vi "Load Selection.vi"() -> ()   [LabVIEW 2020]
panel:
  in  "stop":bool
  in  "12kW Load Bank with 10 Step Control":bool
  in  "1kW Load Bank with 6 Step Control":bool
  # "IoT Programmable Variable Resistive Load Bank"
  # "Select Required Capacity of Load"
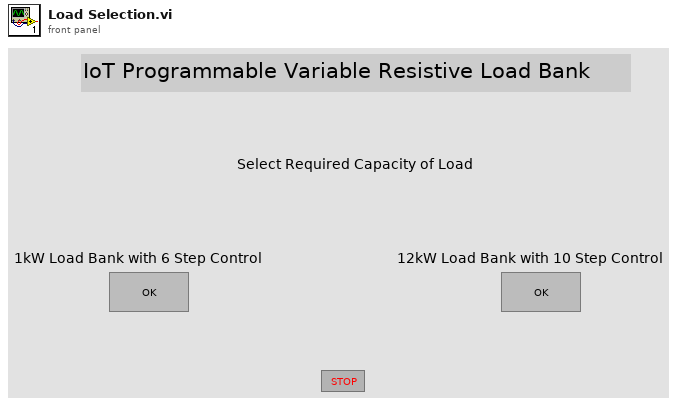
[diagram p1: front panel]
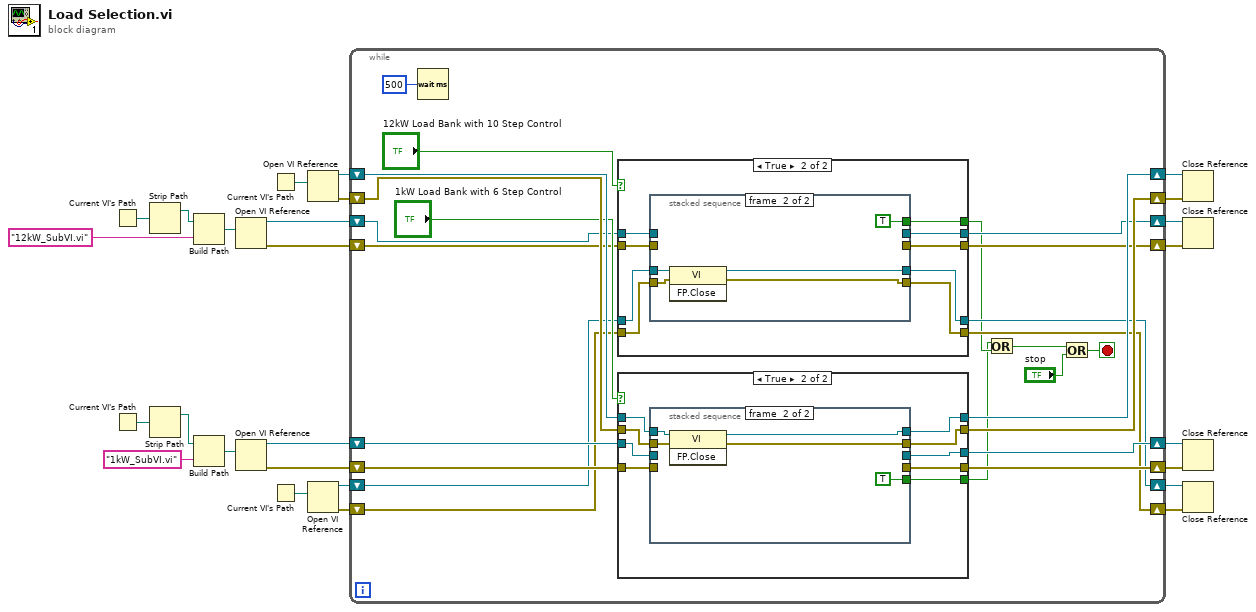
[diagram p0: block diagram]
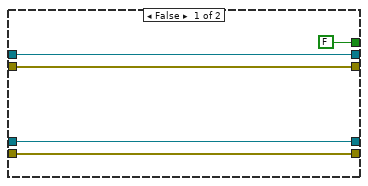
[diagram p2: hidden frame]
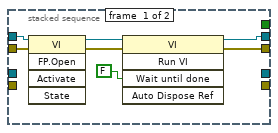
[diagram p3: hidden frame]
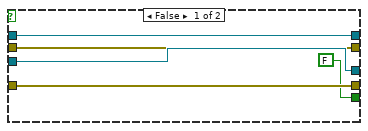
[diagram p4: hidden frame]
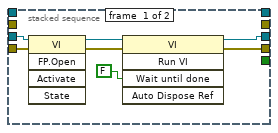
[diagram p5: hidden frame]
diagram:
  n1 = Current VI's Path() -> (path=w9:path)
  n2 = Current VI's Path() -> (path=w26:path)
  n3 = Strip Path(path=w9) -> (stripped path=w8:path)  [unwired: 1 out]
  n4 = Strip Path(path=w26) -> (stripped path=w25:path)  [unwired: 1 out]
  n5 = Build Path(base path=w8, name or relative path="12kW_SubVI.vi") -> (appended path=w7:path)
  n6 = Build Path(base path=w25, name or relative path="1kW_SubVI.vi") -> (appended path=w23:path)
  n7 = Open VI Reference(vi path=w7) -> (vi reference=w1:refnum<vi>, error out=w2:errorcluster)  [unwired: 5 in]
  n8 = Open VI Reference(vi path=w23) -> (vi reference=w22:refnum<vi>, error out=w21:errorcluster)  [unwired: 5 in]
  n9 = Current VI's Path() -> (path=w14:path)
  n10 = Current VI's Path() -> (path=w6:path)
  n11 = Open VI Reference(vi path=w14) -> (vi reference=w18:refnum<vi>, error out=w17:errorcluster)  [unwired: 5 in]
  n12 = Open VI Reference(vi path=w6) -> (vi reference=w3:refnum<vi>, error out=w4:errorcluster)  [unwired: 5 in]
  n13 = while {
    shift-right: [w47] -> w19
    shift-left: w22 -> [w49]
    shift-right: [w46] -> w20
    shift-left: w21 -> [w48]
    shift-right: [w43] -> w16
    shift-left: w18 -> [w45]
    shift-right: [w42] -> w15
    shift-left: w17 -> [w44]
    shift-right: [w37] -> w12
    shift-left: w3 -> [w33]
    shift-right: [w35] -> w10
    shift-left: w1 -> [w31]
    shift-right: [w38] -> w13
    shift-left: w4 -> [w34]
    shift-right: [w36] -> w11
    shift-left: w2 -> [w32]
    stop <- w41 stop-if-true
    n14 = Wait (ms)(milliseconds to wait=u32 500) -> ()  [unwired: 1 out]
    n15 = case shown="True" "12kW Load Bank with 10 Step Control" {
      tunnel: w31 -> [w55 w64]
      tunnel: w32 -> [w54 w63]
      tunnel: [w55 w62] -> w35
      tunnel: [w54 w61] -> w36
      tunnel: w33 -> [w53 w60]
      tunnel: w34 -> [w52 w59]
      tunnel: [w53 w58] -> w37
      tunnel: [w52 w57] -> w38
      tunnel: [FALSE w56] -> w29
      frame False {
      }
      frame True {
        n16 = stacked-sequence {
          tunnel: w64 -> [w71 _]
          tunnel: w63 -> [w70 _]
          tunnel: [w67 _] -> w62
          tunnel: [w66 _] -> w61
          tunnel: w60 -> [_ w76]
          tunnel: w59 -> [_ w75]
          tunnel: [_ w74] -> w58
          tunnel: [_ w72] -> w57
          tunnel: [_ TRUE] -> w56
          frame #0 {
            n17 = invoke class="VI" method="FP.Open"(reference=w71, error in=w70) -> (reference out=w69:refnum<vi>, error out=w68:errorcluster)  [unwired: 3 in, 3 out]
            n18 = invoke class="VI" method="Run VI"(reference=w69, error in=w68, "Wait until done"=FALSE) -> (reference out=w67:refnum<vi>, error out=w66:errorcluster)  [unwired: 2 in, 3 out]
          }
          frame #1 {
            n19 = invoke class="VI" method="FP.Close"(reference=w76, error in=w75) -> (reference out=w74:refnum<vi>, error out=w72:errorcluster)  [unwired: 1 in, 1 out]
          }
        }
      }
    }
    n20 = case shown="True" "1kW Load Bank with 6 Step Control" {
      tunnel: w49 -> [w81 w90]
      tunnel: w48 -> [w80 w89]
      tunnel: [w81 w88] -> w47
      tunnel: [w80 w87] -> w46
      tunnel: w45 -> [w79 w86]
      tunnel: w44 -> [w78 w85]
      tunnel: [w79 w84] -> w43
      tunnel: [w78 w83] -> w42
      tunnel: [FALSE w82] -> w28
      frame False {
      }
      frame True {
        n21 = stacked-sequence {
          tunnel: w90 -> [w97 _]
          tunnel: w89 -> [w96 _]
          tunnel: [w93 _] -> w88
          tunnel: [w92 _] -> w87
          tunnel: w86 -> [_ w102]
          tunnel: w85 -> [_ w101]
          tunnel: [_ w100] -> w84
          tunnel: [_ w98] -> w83
          tunnel: [_ TRUE] -> w82
          frame #0 {
            n22 = invoke class="VI" method="FP.Open"(reference=w97, error in=w96) -> (reference out=w95:refnum<vi>, error out=w94:errorcluster)  [unwired: 3 in, 3 out]
            n23 = invoke class="VI" method="Run VI"(reference=w95, error in=w94, "Wait until done"=FALSE) -> (reference out=w93:refnum<vi>, error out=w92:errorcluster)  [unwired: 2 in, 3 out]
          }
          frame #1 {
            n24 = invoke class="VI" method="FP.Close"(reference=w102, error in=w101) -> (reference out=w100:refnum<vi>, error out=w98:errorcluster)  [unwired: 1 in, 1 out]
          }
        }
      }
    }
    n25 = Or(x=w28, y=w29) -> (x .or. y?=w27:bool)
    n26 = Or(x=w27, y="stop") -> (x .or. y?=w41:bool)
  }
  n27 = Close Reference(reference=w16, error in (no error)=w15) -> ()  [unwired: 1 out]
  n28 = Close Reference(reference=w10, error in (no error)=w11) -> ()  [unwired: 1 out]
  n29 = Close Reference(reference=w19, error in (no error)=w20) -> ()  [unwired: 1 out]
  n30 = Close Reference(reference=w12, error in (no error)=w13) -> ()  [unwired: 1 out]
